vi "Host_FPGA.vi"() -> ()   [LabVIEW 2019]
uses:
  <vilib>/FPGAPlugInAG/myRIO-1900/niLvFpga_Open_myRIO-1900.vi
  <vilib>/rvi/interface/common/dynamic/niFpgaDynamicAddResources.vi
  <vilib>/rvi/interface/common/niFpgaWaitOnOcc.vi
  <vilib>/Utility/error.llb/Error Cluster From Error Code.vi
  <vilib>/rvi/errors/niLvFpgaAdjustHostInterfaceError.vi
  <vilib>/Utility/file.llb/Write Delimited Spreadsheet (I64).vi
  <vilib>/FPGAPlugInAG/Dynamic/niLvFpga_Close_Dynamic.vi
  <vilib>/rvi/interface/nirviOpenFPGA/nirviOpenFPGA.xnode
  FPGA Bitfiles/myriofpga_FPGATarget_MyRIOFPGA_mFGupWJiCJ4.lvbitx
  MyRIO_FPGA.vi
  <vilib>/rvi/interface/nirviMethod/nirviMethod.xnode
  <vilib>/rvi/interface/nirviReadWriteControl/nirviReadWriteControl.xnode
  <vilib>/rvi/interface/nirviCloseFPGA/nirviCloseFPGA.xnode
  <vilib>/rvi/errors/niLvFpgaMergeErrorWithErrorCode.vi
  <vilib>/FPGAPlugInAG/Dynamic/niLvFpga_ReadFifo_Dynamic.vi
  <vilib>/FPGAPlugInAG/Dynamic/niLvFpga_ConfigureFifo_Dynamic.vi
  NiFpgaLv.dll
  <vilib>/rvi/interface/Simulation/niFpgaSimulationCallBeginRW.vi
  <vilib>/FPGAPlugInAG/Dynamic/niLvFpga_StopFifo_Dynamic.vi
panel:
  out "Waveform Chart 3":i16[](graph)
  out "Waveform Chart 2":i16[](graph)
  out "Waveform Chart":i16[](graph)
  in  "file path (dialog if empty)":path
  in  "OK Button":bool
  out "Actual Depth":u32
  out "Data in Volts":dbl[][](graph)
  out "loop time":u32
  in  "FPGA loop timer (us)":u32=1000
  out "error out":errorcluster
  in  "milliseconds to wait":u32=100
  in  "stop":bool
  out "Data to Read":u32[](graph)
  out "Data":i16[][](graph)
  # "Buffer size 10000 points on PC\nRead data in blocks of 4096 points\n4 channels so 1024 points per channel"
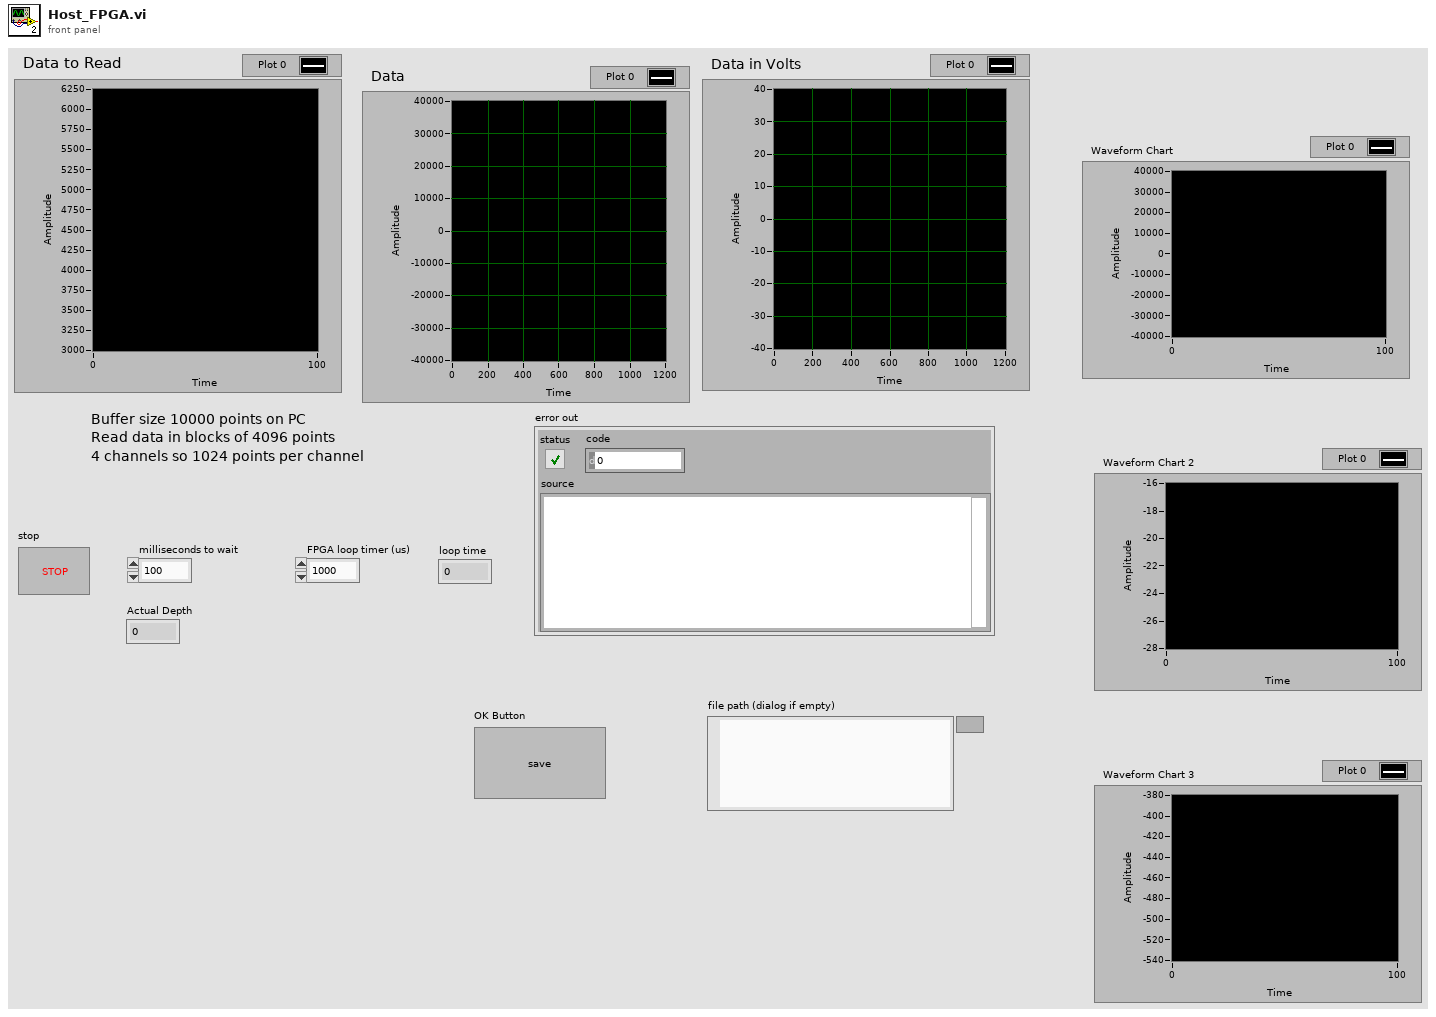
[diagram p1: front panel]
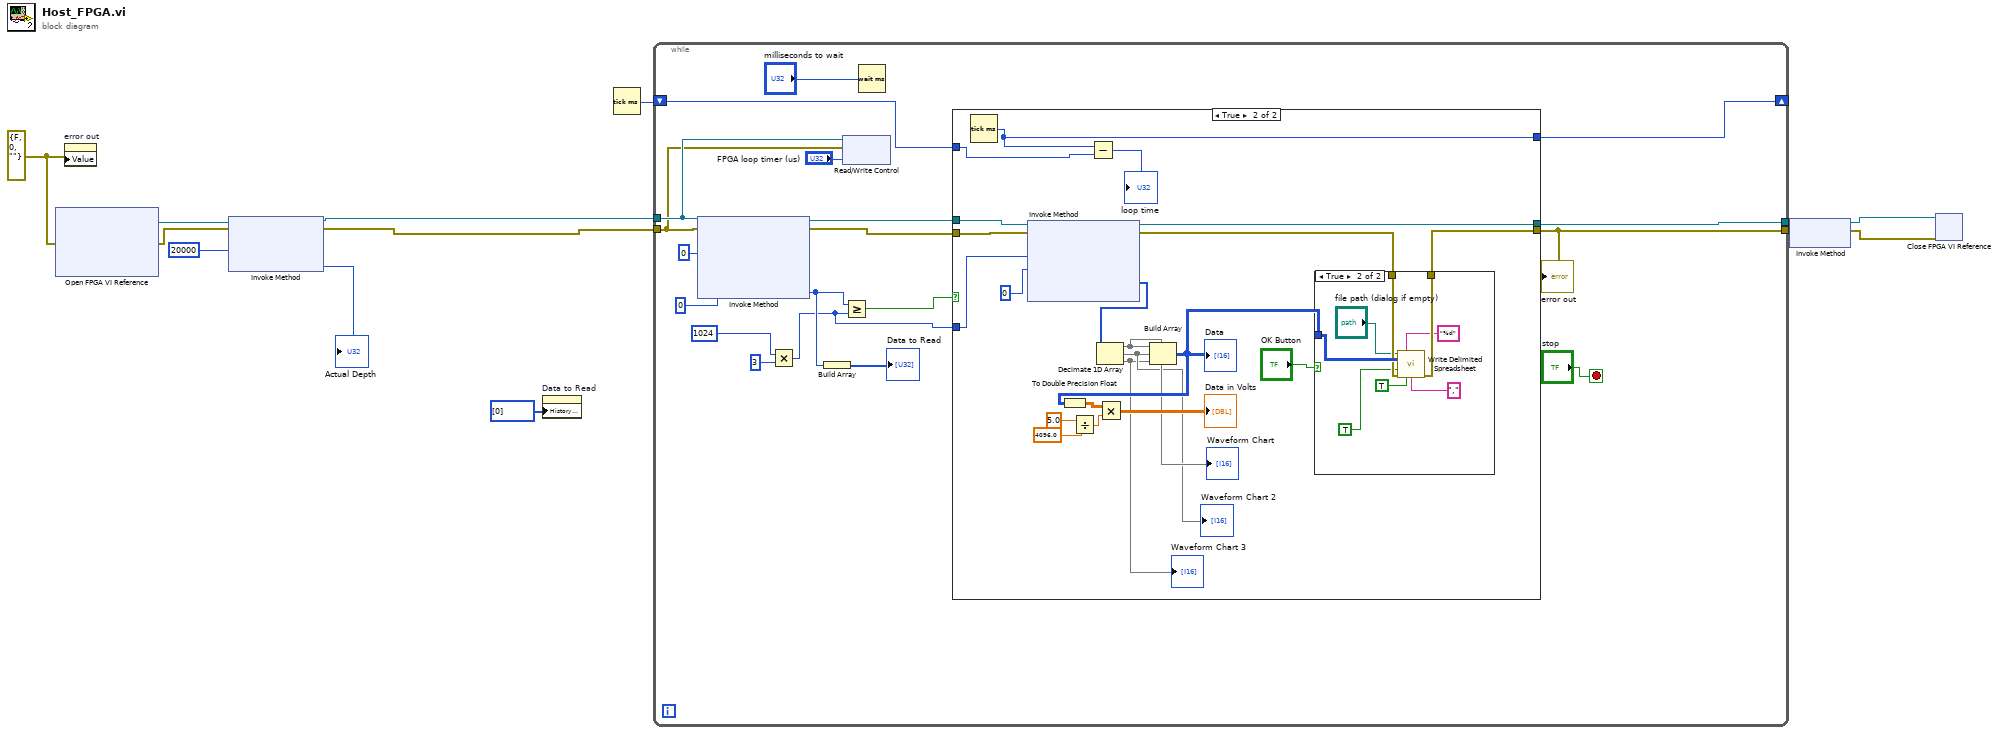
[diagram p0: block diagram]
diagram:
  w11 = errorcluster {"status"=FALSE, "code"=0, "source"=""} ("error constant")
  n1 = xnode "Open FPGA VI Reference"("error in"=w11) -> ("FPGA VI Reference Out"=w5:refnum<k20>, "error out"=w4:errorcluster)  [unwired: 1 in]
  n2 = property on="error out" class="Clust (strict)"("Value"=w11) -> ()  [unwired: 2 in, 2 out]
  n3 = xnode "Invoke Method"("FPGA VI Reference In"=w5, "error in"=w4, "Requested Depth"=u32 20000) -> ("FPGA VI Reference Out"=w2:refnum<k20>, "error out"=w1:errorcluster, "Actual Depth"=→"Actual Depth":u32)
  n4 = property on="Data to Read" class="WFChart (strict)"("History Data"=u32[] [0]) -> ()  [unwired: 2 in, 2 out]
  n5 = Tick Count (ms)() -> (millisecond timer value=w10:u32)
  n6 = while {
    tunnel: w2 -> [w25]
    tunnel: w1 -> [w24]
    tunnel: [w27] -> w9
    tunnel: [w26] -> w8
    shift-right: [w22] -> _
    shift-left: w10 -> [w23]
    stop <- "stop" stop-if-true
    n7 = xnode "Invoke Method"("FPGA VI Reference In"=w25, "error in"=w24, "Number of Elements"=u32 0, "Timeout (ms)"=0) -> ("FPGA VI Reference Out"=w31:refnum<k20>, "error out"=w30:errorcluster, "Elements Remaining"=w17:u32)  [unwired: 1 out]
    n8 = Multiply(x=u32 1024 ("y"), y=u32 3) -> (x*y=w14:u32)
    n9 = Build Array(w17) -> (→"Data to Read":u32[])
    n10 = xnode "Read/Write Control"("FPGA VI Reference In"=w25, "error in"=w24, "timer"="FPGA loop timer (us)") -> ()  [unwired: 2 out]
    n11 = Greater Or Equal?(x=w17, y=w14) -> (x >= y?=w32:bool)
    n12 = Wait (ms)(milliseconds to wait="milliseconds to wait") -> ()  [unwired: 1 out]
    n13 = case shown="True" w32 {
      tunnel: w31 -> [w35 w56]
      tunnel: w30 -> [w34 w55]
      tunnel: w14 -> [_ w44]
      tunnel: [w35 w53] -> w26
      tunnel: [w34 w39] -> w27
      tunnel: w23 -> [w33 w52]
      tunnel: [w33 w50] -> w22
      frame False {
      }
      frame True {
        n14 = Tick Count (ms)() -> (millisecond timer value=w50:u32)
        n15 = xnode "Invoke Method"("FPGA VI Reference In"=w56, "error in"=w55, "Number of Elements"=w44, "Timeout (ms)"=0) -> ("FPGA VI Reference Out"=w53:refnum<k20>, "error out"=w40:errorcluster, "Data"=w54:i16[])  [unwired: 1 out]
        n16 = Divide(x=5.0, y=4096.0) -> (x/y=w48:dbl)
        n17 = Subtract(x=w50, y=w52) -> (x-y=→"loop time":u32)
        n18 = Decimate 1D Array "Decimate 1D Array"(w54) -> (w38:i16[], w37:i16[], w36:i16[])
        "Waveform Chart" <- w38
        "Waveform Chart 2" <- w37
        "Waveform Chart 3" <- w36
        n19 = Build Array(w38, w37, w36) -> (w41:i16[][])
        "Data" <- w41
        n20 = To Double Precision Float(number=w41) -> (double precision float=w49:dbl[][])
        n21 = Multiply(x=w49, y=w48) -> (x*y=→"Data in Volts":dbl[][])
        n22 = case shown="True" "OK Button" {
          tunnel: w41 -> [_ w65]
          tunnel: w40 -> [w57 w64]
          tunnel: [w57 w62] -> w39
          frame False {
          }
          frame True {
            n23 = call-poly <vilib>:"Write Delimited Spreadsheet.vi"("file path (dialog if empty)"="file path (dialog if empty)", "format (%d)"="%d", "2D data"=w65, "append to file? (new file:F)"=TRUE, "error in (no error)"=w64, "transpose? (no:F)"=TRUE, "delimiter (\\t)"="," ("delimiter (\\t)")) -> ("error out"=w62:errorcluster)  [unwired: 7 in, 1 out]
          }
        }
      }
    }
    "error out" <- w27
  }
  n24 = xnode "Invoke Method"("FPGA VI Reference In"=w8, "error in"=w9) -> ("FPGA VI Reference Out"=w12:refnum<k20>, "error out"=w13:errorcluster)
  n25 = xnode "Close FPGA VI Reference"("FPGA VI Reference In"=w12, "error in"=w13) -> ()  [unwired: 1 out]
